vi "Unwield.vi"(8 "Error In":errorcluster, 11 "reference in":refnum<class "Hammer.lvclass">) -> (0 "Error Out":errorcluster, 3 "reference out":refnum<class "Hammer.lvclass">)   [LabVIEW 2020, in "Hammer.lvclass"]
uses:
  Hammer.lvclass
  IEnchantment_interface/IEnchantment.lvclass
  Console_class/Console.lvclass
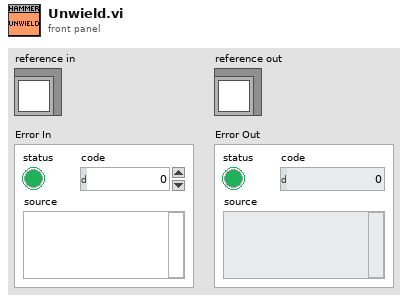
[diagram p1: front panel]
types:
  T1 = typedef "Hammer.lvclass/ObjectAttributes.ctl" = cluster{"_enchantment":refnum<class "IEnchantment.lvclass">}
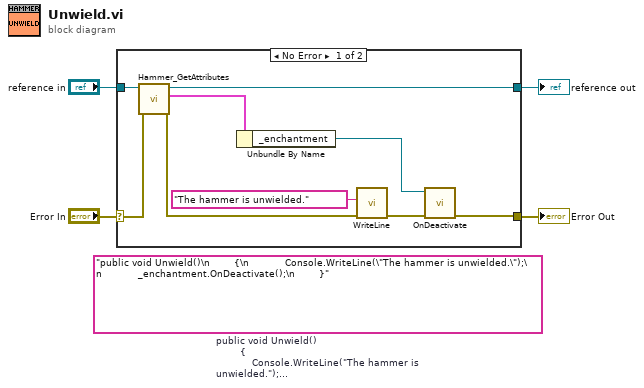
[diagram p0: block diagram]
diagram:
  (unwired) "public void Unwield()\n        {\n            Console.WriteLine(\"The hammer is unwielded.\");\n            _enchantment.OnDeactivate();\n        }"  # public void Unwield()         {             Console.WriteLine("The hammer is unwielded.");             _enchantment.OnDeactivate();         }
  n1 = case shown="No Error" "Error In" {
    selector: "Error In" -> [w7 w15]
    tunnel: [w6 w15] -> w3
    tunnel: [w5 w14] -> w1
    tunnel: "reference in" -> [w8 w14]
    frame No Error {
      n2 = call "Hammer_GetAttributes.vi"("error in (no error)"=w7, "reference in"=w8) -> ("error out"=w9:errorcluster, "Data"=w10:T1, "reference out"=w5:refnum<class "Hammer.lvclass">)  [unwired: 6 in, 1 out]
      n3 = Unbundle By Name(w10) -> ("_enchantment"=w13:refnum<class "IEnchantment.lvclass">)
      n4 = call "WriteLine.vi"("Error In"=w9, "ConsoleText"="The hammer is unwielded.") -> ("Error Out"=w11:errorcluster)  [unwired: 9 in]
      n5 = call-dynamic "OnDeactivate.vi"("Error In"=w11, "object in"=w13) -> ("Error Out"=w6:errorcluster)  [unwired: 8 in, 1 out]
    }
    frame Error {
    }
  }
  "Error Out" <- w3
  "reference out" <- w1
